vi "PPG_ABC.calc pattern times.vi"(0 "i ref in":refnum<vi>, 1 "channelTimes":dbl[][](array[numeric]), 5 "error in (no error)":errorcluster) -> (14 "i ref out":refnum<vi>, 15 "patternTimes":dbl[](array[numeric]), 16 "patterns":u64[](array[numeric]), 19 "error out":errorcluster)   [LabVIEW 2014, in "PPG_ABC.lvlib"]
doc: "Calculates the output patterns together with the absolute times, at which the patterns are to be applied."
uses:
  PPG_ABC.lvlib
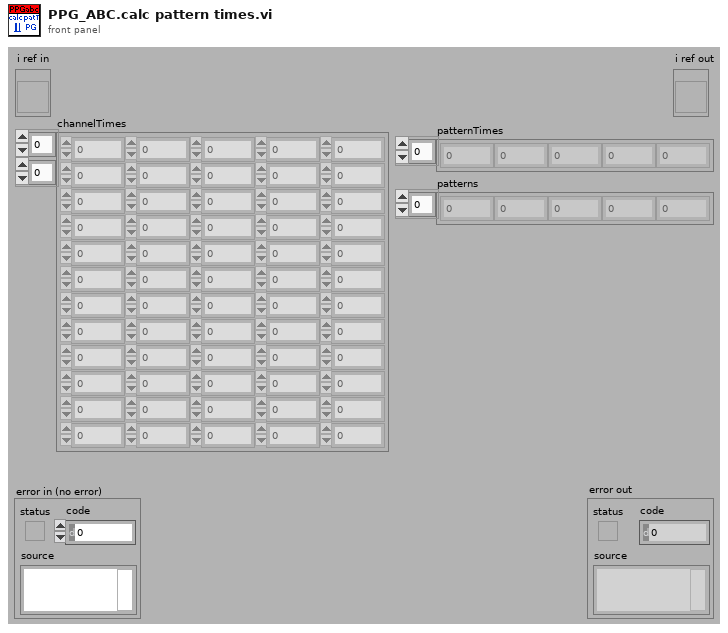
[diagram p1: front panel]
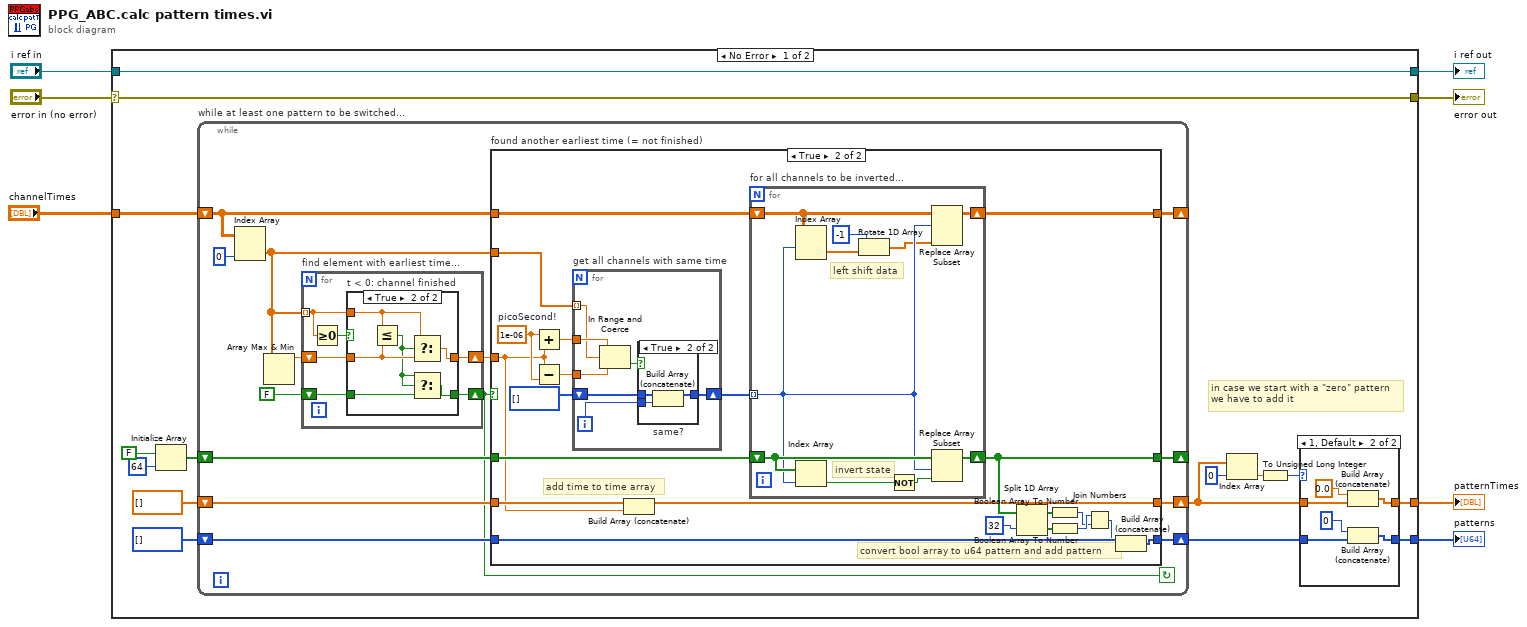
[diagram p0: block diagram]
diagram:
  n1 = case shown="No Error" "error in (no error)" {
    selector: "error in (no error)" -> [w21 w105]
    tunnel: "i ref in" -> [w22 w106]
    tunnel: [w22 w106] -> w6
    tunnel: [w21 w105] -> w5
    tunnel: "channelTimes" -> [w16 _]
    tunnel: [w10 _] -> w2
    tunnel: [w8 _] -> w1
    frame No Error {
      # "in case we start with a \"zero\" pattern\nwe have to add it"
      n2 = Initialize Array(FALSE, 64 ("dimension size")) -> (w18:bool[])
      n3 = while "while at least one pattern to be switched..." {
        shift-right: [w37] -> _
        shift-left: w18 -> [w43]
        shift-right: [w39] -> _
        shift-left: w16 -> [w42]
        shift-right: [w40] -> w11
        shift-left: dbl[] [] -> [w41]
        shift-right: [w34] -> w9
        shift-left: u64[] [] -> [w35]
        stop <- w33 continue-if-true
        n4 = Index Array(array=w42, index (col)=0 ("index (row)")) -> (element=w32:dbl[])  [unwired: 1 in]
        n5 = Array Max & Min(array=w32) -> (max value=w31:dbl)  [unwired: 3 out]
        n6 = for "find element with earliest time..." {
          tunnel: w32 -> [w95] mode=indexing
          shift-right: [w92] -> w33
          shift-left: FALSE -> [w93]
          shift-right: [w91] -> w44
          shift-left: w31 -> [w94]
          n7 = Greater Or Equal To 0?(x=w95) -> (x >= 0?=w96:bool)
          n8 = case "t < 0: channel finished" shown="True" w96 {
            tunnel: w95 -> [_ w100]
            tunnel: w94 -> [w97 w101]
            tunnel: w93 -> [w98 w104]
            tunnel: [w98 w103] -> w92
            tunnel: [w97 w102] -> w91
            frame False {
            }
            frame True {
              n9 = Less Or Equal?(x=w100, y=w101) -> (x <= y?=w99:bool)
              n10 = Select(t=w100, s=w99, f=w101) -> (s? t:f=w102:dbl)
              n11 = Select(t=w99, s=w99, f=w104) -> (s? t:f=w103:bool)
            }
          }
        }
        n12 = case "found another earliest time (= not finished)" shown="True" w33 {
          tunnel: w44 -> [_ w51]
          tunnel: w32 -> [_ w69]
          tunnel: w43 -> [w47 w64]
          tunnel: w42 -> [w48 w63]
          tunnel: w41 -> [w46 w52]
          tunnel: [w46 w53] -> w40
          tunnel: [w48 w62] -> w39
          tunnel: [w47 w57] -> w37
          tunnel: w35 -> [w45 w56]
          tunnel: [w45 w55] -> w34
          frame False {
          }
          frame True {
            w65 = 1e-06  # picoSecond!
            # "add time to time array"
            # "convert bool array to u64 pattern and add pattern"
            n13 = Add(x=w65, y=w51) -> (x+y=w68:dbl)
            n14 = Subtract(x=w51, y=w65) -> (x-y=w67:dbl)
            n15 = for "get all channels with same time" {
              shift-right: [w81] -> w61
              shift-left: i32[] [] -> [w82]
              tunnel: w69 -> [w84] mode=indexing
              tunnel: w68 -> [w86]
              tunnel: w67 -> [w85]
              i -> [w80]
              n16 = In Range and Coerce(upper limit=w86, x=w84, lower limit=w85) -> (In Range?=w83:bool)  [unwired: 1 out]
              n17 = case "same?" shown="True" w83 {
                tunnel: w82 -> [w87 w90]
                tunnel: [w87 w89] -> w81
                tunnel: w80 -> [_ w88]
                frame False {
                }
                frame True {
                  n18 = Build Array (concatenate)(w90, w88) -> (w89:i32[])
                }
              }
            }
            n19 = Build Array (concatenate)(w52, w51) -> (w53:dbl[])
            n20 = for "for all channels to be inverted..." {
              tunnel: w61 -> [w74] mode=indexing
              shift-right: [w75] -> w62
              shift-left: w63 -> [w76]
              shift-right: [w73] -> w57
              shift-left: w64 -> [w79]
              # "invert state"
              # "left shift data"
              n21 = Index Array(array=w76, index (row)=w74) -> (element=w72:dbl[])  [unwired: 1 in]
              n22 = Index Array(array=w79, index=w74) -> (element=w78:bool)
              n23 = Rotate 1D Array(1:w72, 2:-1 ("n")) -> (0:w71:dbl[])
              n24 = Not(x=w78) -> (.not. x?=w77:bool)
              n25 = Replace Array Subset(array=w76, new element=w71, index (row)=w74) -> (w75:dbl[][])  [unwired: 1 in]
              n26 = Replace Array Subset(array=w79, new element=w77, index=w74) -> (w73:bool[])
            }
            n27 = Split 1D Array(array=w57, index=32) -> (first subarray=w59:bool[], second subarray=w58:bool[])
            n28 = Boolean Array To Number(Boolean array=w59) -> (number=w49:u32)
            n29 = Boolean Array To Number(Boolean array=w58) -> (number=w50:u32)
            n30 = Join Numbers(hi=w50, lo=w49) -> ((hi.lo)=w54:u64)
            n31 = Build Array (concatenate)(w56, w54) -> (w55:u64[])
          }
        }
      }
      n32 = Index Array(array=w11, index=0) -> (element=w13:dbl)
      n33 = To Unsigned Long Integer(number=w13) -> (unsigned 32bit integer=w12:u32)
      n34 = case shown="1, Default" w12 {
        tunnel: w11 -> [w24 w28]
        tunnel: [w24 w30] -> w10
        tunnel: w9 -> [w23 w26]
        tunnel: [w23 w29] -> w8
        frame 0 {
        }
        frame 1, Default {
          n35 = Build Array (concatenate)(0.0, w28) -> (w30:dbl[])
          n36 = Build Array (concatenate)(u64 0, w26) -> (w29:u64[])
        }
      }
    }
    frame Error {
    }
  }
  "error out" <- w5
  "i ref out" <- w6
  "patternTimes" <- w2
  "patterns" <- w1
